vi "Get Scene Data.vi"(6 "Control Ref Queue":T6, 7 "Multiplot Representation In":T3, 8 "error in (no error)":errorcluster, 9 "Data In":refnum<class "3D Plot Datatype.lvclass">[](array[class]), 10 "Actual Transform In":T1, 11 "3D Plot.lvclass in":refnum<class "3D Plot.lvclass">) -> (0 "error out":errorcluster, 1 "Data Out":refnum<class "3D Plot Datatype.lvclass">[](array[class]), 2 "Actual Transform Out":T1, 3 "3D Plot.lvclass out":refnum<class "3D Plot.lvclass">, 4 "Data Cleaned?":bool, 5 "Multiplot Representation Out":T3)   [LabVIEW 2020, in "3D Plot.lvclass"]
uses:
  3D Plot.lvclass
  3DMathPlot Ctrl Act Queue.ctl
  3DMathPlot Ctrl Act Cluster.ctl
  3DMathPlot State Class.ctl
  3D Plot Datatype.lvclass
  Multiplot Representation.ctl
  Plot Representation.ctl
  Range Clusters.ctl
  Mesh Data.ctl
  Actual Transform.ctl
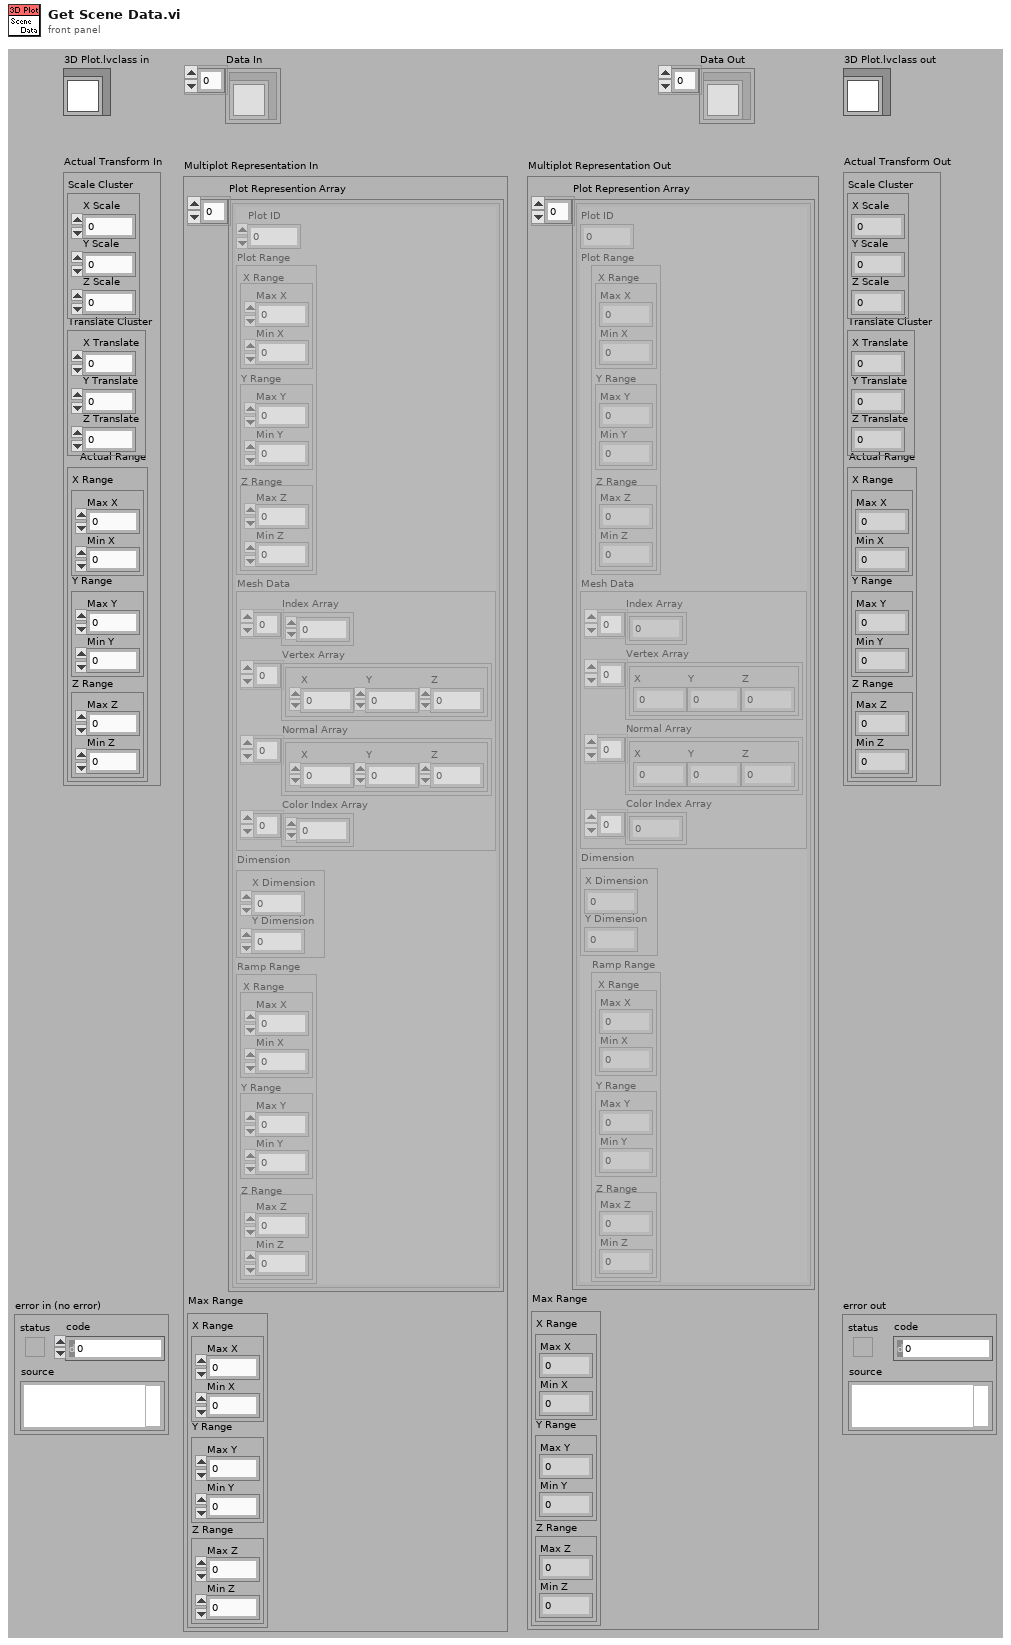
[diagram p1: front panel]
types:
  T1 = typedef "3D Plot.lvclass/Actual Transform.ctl" = cluster{"Scale Cluster":cluster{"X Scale":sgl, "Y Scale":sgl, "Z Scale":sgl}, "Translate Cluster":cluster{"X Translate":sgl, "Y Translate":sgl, "Z Translate":sgl}, "Actual Range":T2}
  T2 = typedef "3D Plot.lvclass/Range Clusters.ctl" = cluster{"X Range":cluster{"Max X":sgl, "Min X":sgl}, "Y Range":cluster{"Max Y":sgl, "Min Y":sgl}, "Z Range":cluster{"Max Z":sgl, "Min Z":sgl}}
  T3 = typedef "3D Plot.lvclass/Multiplot Representation.ctl" = cluster{"Plot Represention Array":T4[], "Max Range":T2}
  T4 = typedef "3D Plot.lvclass/Plot Representation.ctl" = cluster{"Plot ID":i32, "Plot Range":T2, "Mesh Data":T5, "Dimension":cluster{"X Dimension":i32, "Y Dimension":i32}, "Ramp Range":T2}
  T5 = typedef "3D Plot.lvclass/Mesh Data.ctl" = cluster{"Index Array":u32[], "Vertex Array":cluster{"X":sgl, "Y":sgl, "Z":sgl}[], "Normal Array":cluster{"X":sgl, "Y":sgl, "Z":sgl}[], "Color Index Array":i32[]}
  T6 = typedef "3DMathPlot Ctrl Act Queue.ctl" = refnum<queue>
  T7 = typedef "3DMathPlot Ctrl Act Cluster.ctl" = cluster{"3D Picture Control":refnum<vi>, "Render Window Refnum":refnum<vi>, "XY Graph":refnum<vi>, "Intensity Graph":refnum<vi>, "Color Legend Palette":refnum<vi>, "Projection Palette":refnum<vi>, "XControl  Ref":refnum<vi>, "Facade Ref":refnum<vi>, "Export Image Ref":refnum<vi>, "Clear Data Flag":bool, "Display State Change Class":T8}
  T8 = typedef "3DMathPlot State Class.ctl" = enum16{"Update All Objects (Undo)", "Update Light Object Only", "Update Axis Object Only", "Update Plot Object Only", "Update Cursor Object Only", "Update Axis Plot Cursor Objects", "No Update"}
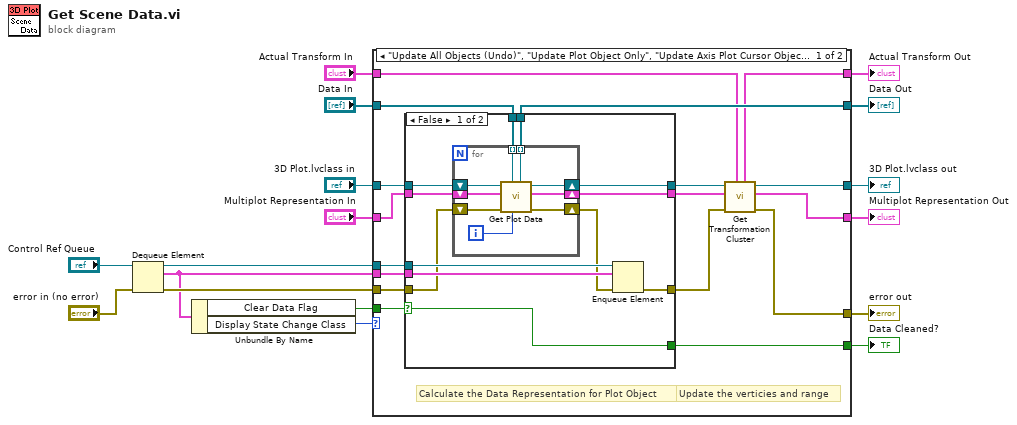
[diagram p0: block diagram]
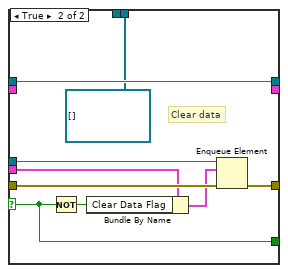
[diagram p2: hidden frame]
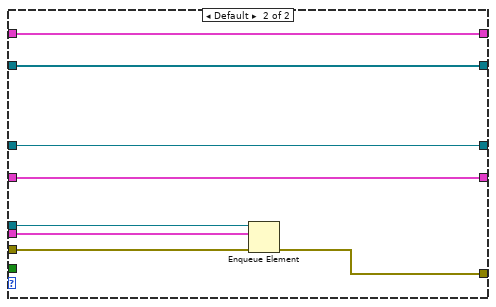
[diagram p3: hidden frame]
diagram:
  n1 = Dequeue Element(queue="Control Ref Queue", error in (no error)="error in (no error)") -> (queue out=w5:T6, element=w6:T7, error out=w7:errorcluster)  [unwired: 2 out]
  n2 = Unbundle By Name(w6) -> ("Clear Data Flag"=w4:bool, "Display State Change Class"=w1:T8)
  n3 = case shown="\"Update All Objects (Undo)\", \"Update Plot Object Only\", \"Update Axis Plot Cursor Objects\"" w1 {
    tunnel: "3D Plot.lvclass in" -> [w34 w70]
    tunnel: [w33 _] -> w16
    tunnel: "Data In" -> [w32 w71]
    tunnel: "Multiplot Representation In" -> [w31 w69]
    tunnel: [w30 w71] -> w13
    tunnel: [w29 w66] -> w12
    tunnel: [w28 w70] -> w11
    tunnel: [w27 w69] -> w10
    tunnel: [w26 w72] -> w9
    tunnel: "Actual Transform In" -> [w25 w72]
    tunnel: w7 -> [w24 w65]
    tunnel: w6 -> [w23 w67]
    tunnel: w5 -> [w22 w68]
    tunnel: w4 -> [w21 _]
    frame "Update All Objects (Undo)", "Update Plot Object Only", "Update Axis Plot Cursor Objects" {
      # "Update the verticies and range"
      # "Calculate the Data Representation for Plot Object"
      n4 = case shown="False" w21 {
        selector: w21 -> [w35 w56]
        tunnel: [w46 refnum<class "3D Plot Datatype.lvclass">[] []] -> w30
        tunnel: w31 -> [w45 _]
        tunnel: [w44 _] -> w18
        tunnel: [w37 w60] -> w20
        tunnel: w24 -> [w36 w61]
        tunnel: w32 -> [w43 _]
        tunnel: w34 -> [w42 w64]
        tunnel: [w41 w64] -> w19
        tunnel: [w35 w56] -> w33
        tunnel: w22 -> [w40 w62]
        tunnel: w23 -> [w39 w59]
        frame False {
          n5 = for {
            tunnel: w43 -> [w55] mode=indexing
            tunnel: [w54] -> w46 mode=indexing
            shift-right: [w52] -> w38
            shift-left: w36 -> [w50]
            shift-right: [w51] -> w44
            shift-left: w45 -> [w53]
            shift-right: [w47] -> w41
            shift-left: w42 -> [w48]
            i -> [w49]
            n6 = call "Get Plot Data.vi"("Index"=w49, "3D Plot Datatype.lvclass in"=w55, "error in (no error)"=w50, "Plot Representation In"=w53, "3D Plot.lvclass in"=w48) -> ("error out"=w52:errorcluster, "Plot Representation Out"=w51:T3, "3D Plot.lvclass out"=w47:refnum<class "3D Plot.lvclass">, "3D Plot Datatype.lvclass out"=w54:refnum<class "3D Plot Datatype.lvclass">)  [unwired: 3 out]
          }
          n7 = Enqueue Element(queue=w40, element=w39, error in (no error)=w38) -> (error out=w37:errorcluster)  [unwired: 3 out]
        }
        frame True {
          # "Clear data"
          n8 = Not(x=w56) -> (.not. x?=w57:bool)
          n9 = Bundle By Name(cluster=w59, "Clear Data Flag"=w57) -> (w58:T7)
          n10 = Enqueue Element(queue=w62, element=w58, error in (no error)=w61) -> (error out=w60:errorcluster)  [unwired: 3 out]
        }
      }
      n11 = call "Get Transformation Cluster.vi"("Actual Transform In"=w25, "error in (no error)"=w20, "Multiplot Representation In"=w18, "3D Plot.lvclass in"=w19) -> ("error out"=w29:errorcluster, "Multiplot Representation Out"=w27:T3, "3D Plot.lvclass out"=w28:refnum<class "3D Plot.lvclass">, "Actual Transform Out"=w26:T1)  [unwired: 4 out]
    }
    frame Default {
      n12 = Enqueue Element(queue=w68, element=w67, error in (no error)=w65) -> (error out=w66:errorcluster)  [unwired: 3 out]
    }
  }
  "3D Plot.lvclass out" <- w11
  "error out" <- w12
  "Data Cleaned?" <- w16
  "Multiplot Representation Out" <- w10
  "Data Out" <- w13
  "Actual Transform Out" <- w9
